vi "Init Range Single.vi"(8 "error in (no error)":errorcluster, 11 "Grove Ranging Sensor VL53L0X in":refnum<class "Grove Range Sensor VL53L0X .lvclass">) -> (0 "error out":errorcluster, 3 "Grove Ranging Sensor VL53L0X out":refnum<class "Grove Range Sensor VL53L0X .lvclass">)   [LabVIEW 2020, in "CTI-Peripheral.lvlib" / "Grove Range Sensor VL53L0X .lvclass"]
uses:
  Grove Range Sensor VL53L0X .lvclass
  Range Mode.ctl
  Sensor Command.ctl
  Registers.ctl
  Grove Range Sensor VL53L0X .lvclass/Grove Range Sensor VL53L0X .ctl
  CTI/I2C Connection/I2C Connection.lvclass/I2C Connection.ctl
  CTI/Session/I2C Write Data.vi
  CTI/Session/I2C Read Data.vi
  CTI/I2C Connection/I2C Connection.lvclass
panel:
  out "Init Data":string
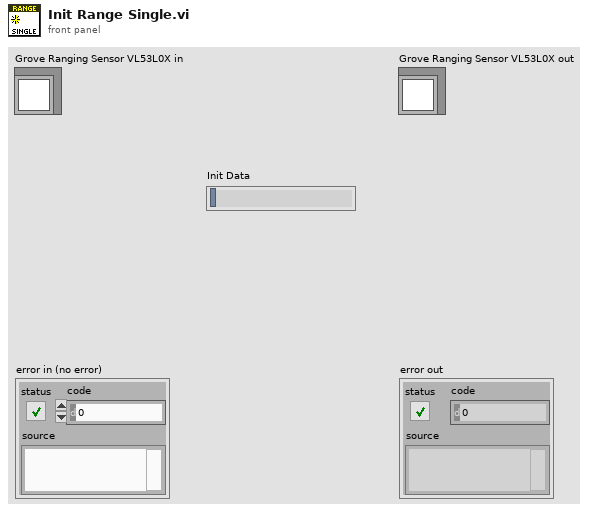
[diagram p1: front panel]
types:
  T1 = typedef "CTI-Peripheral.lvlib/Grove Range Sensor VL53L0X .lvclass/Sensor Command.ctl" = cluster{"Registers":T2, "Data":u8[], "ReadBack Len":u8}
  T2 = typedef "CTI-Peripheral.lvlib/Grove Range Sensor VL53L0X .lvclass/Registers.ctl" = u16
  T3 = typedef "CTI-Peripheral.lvlib/Grove Range Sensor VL53L0X .lvclass/Range Mode.ctl" = enum16{"No Mode - Error", "Single", "Continuous", "High Speed", "High Accuracy", "Long Distance"}
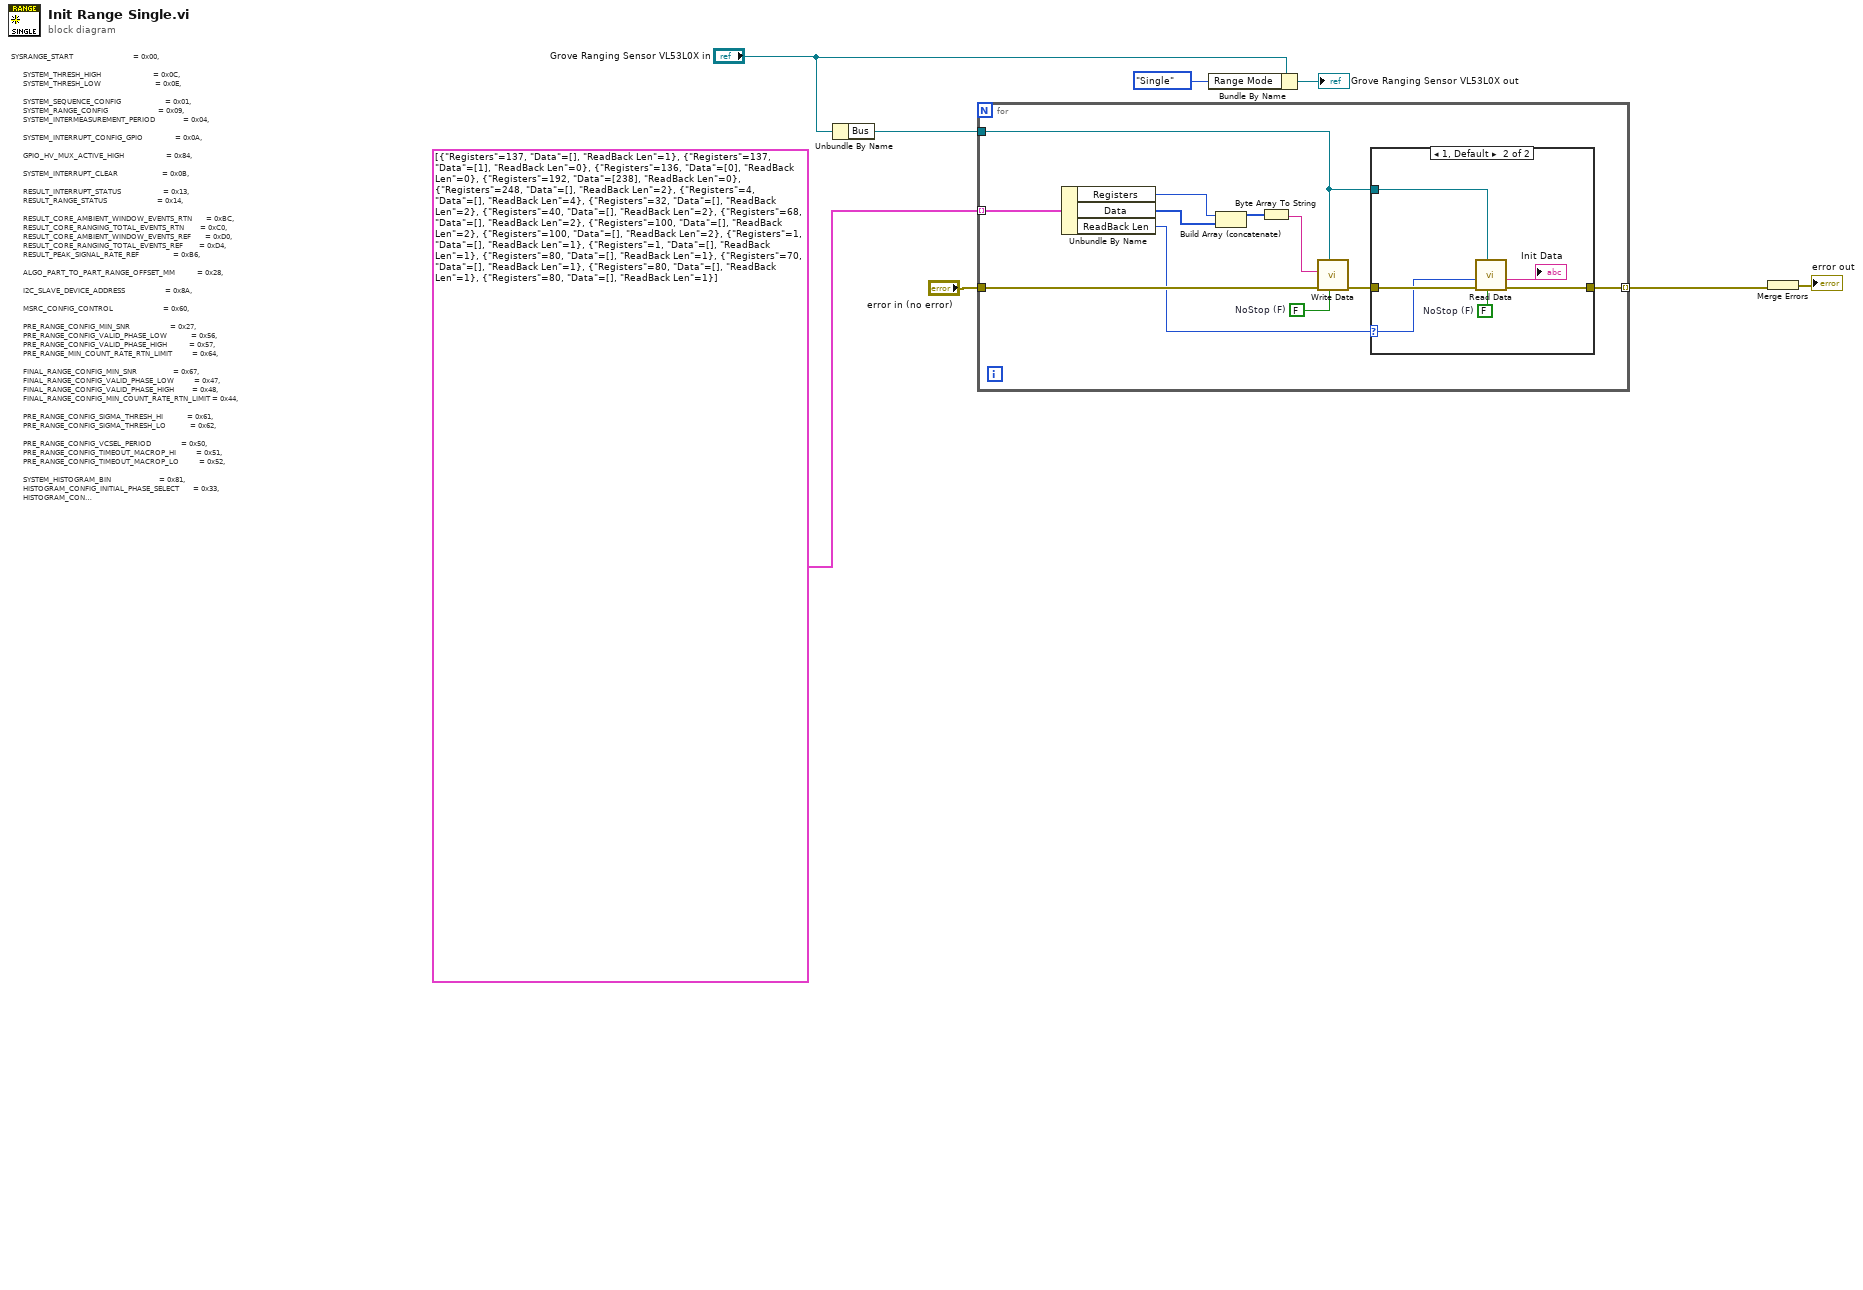
[diagram p0: block diagram]
diagram:
  # "SYSRANGE_START                              = 0x00,\n\n      SYSTEM_THRESH_HIGH                          = 0x0C,\n      SYSTEM_THRESH_LOW                           = 0x0E,\n\n      SYSTEM_SEQUENCE_CONFIG                      = 0x01,\n      SYSTEM_RANGE_CONFIG                         = 0x09,\n      SYSTEM_INTERMEASUREMENT_PERIOD              = 0x04,\n\n      SYSTEM_INTERRUPT_CONFIG_GPIO                = 0x0A,\n\n      GPIO_HV_MUX_ACTIVE_HIGH                     = 0x84,\n\n      SYSTEM_INTERRUPT_CLEAR                      = 0x0B,\n\n      RESULT_INTERRUPT_STATUS                     = 0x13,\n      RESULT_RANGE_STATUS                         = 0x14,\n\n      RESULT_CORE_AMBIENT_WINDOW_EVENTS_RTN       = 0xBC,\n      RESULT_CORE_RANGING_TOTAL_EVENTS_RTN        = 0xC0,\n      RESULT_CORE_AMBIENT_WINDOW_EVENTS_REF       = 0xD0,\n      RESULT_CORE_RANGING_TOTAL_EVENTS_REF        = 0xD4,\n      RESULT_PEAK_SIGNAL_RATE_REF                 = 0xB6,\n\n      ALGO_PART_TO_PART_RANGE_OFFSET_MM           = 0x28,\n\n      I2C_SLAVE_DEVICE_ADDRESS                    = 0x8A,\n\n      MSRC_CONFIG_CONTROL                         = 0x60,\n\n      PRE_RANGE_CONFIG_MIN_SNR                    = 0x27,\n      PRE_RANGE_CONFIG_VALID_PHASE_LOW            = 0x56,\n      PRE_RANGE_CONFIG_VALID_PHASE_HIGH           = 0x57,\n      PRE_RANGE_MIN_COUNT_RATE_RTN_LIMIT          = 0x64,\n\n      FINAL_RANGE_CONFIG_MIN_SNR                  = 0x67,\n      FINAL_RANGE_CONFIG_VALID_PHASE_LOW          = 0x47,\n      FINAL_RANGE_CONFIG_VALID_PHASE_HIGH         = 0x48,\n      FINAL_RANGE_CONFIG_MIN_COUNT_RATE_RTN_LIMIT = 0x44,\n\n      PRE_RANGE_CONFIG_SIGMA_THRESH_HI            = 0x61,\n      PRE_RANGE_CONFIG_SIGMA_THRESH_LO            = 0x62,\n\n      PRE_RANGE_CONFIG_VCSEL_PERIOD               = 0x50,\n      PRE_RANGE_CONFIG_TIMEOUT_MACROP_HI          = 0x51,\n      PRE_RANGE_CONFIG_TIMEOUT_MACROP_LO          = 0x52,\n\n      SYSTEM_HISTOGRAM_BIN                        = 0x81,\n      HISTOGRAM_CONFIG_INITIAL_PHASE_SELECT       = 0x33,\n      HISTOGRAM_CONFIG_READOUT_CTRL               = 0x55,\n\n      FINAL_RANGE_CONFIG_VCSEL_PERIOD             = 0x70,\n      FINAL_RANGE_CONFIG_TIMEOUT_MACROP_HI        = 0x71,\n      FINAL_RANGE_CONFIG_TIMEOUT_MACROP_LO        = 0x72,\n      CROSSTALK_COMPENSATION_PEAK_RATE_MCPS       = 0x20,\n\n      MSRC_CONFIG_TIMEOUT_MACROP                  = 0x46,\n\n      SOFT_RESET_GO2_SOFT_RESET_N                 = 0xBF,\n      IDENTIFICATION_MODEL_ID                     = 0xC0,\n      IDENTIFICATION_REVISION_ID                  = 0xC2,\n\n      OSC_CALIBRATE_VAL                           = 0xF8,\n\n      GLOBAL_CONFIG_VCSEL_WIDTH                   = 0x32,\n      GLOBAL_CONFIG_SPAD_ENABLES_REF_0            = 0xB0,\n      GLOBAL_CONFIG_SPAD_ENABLES_REF_1            = 0xB1,\n      GLOBAL_CONFIG_SPAD_ENABLES_REF_2            = 0xB2,\n      GLOBAL_CONFIG_SPAD_ENABLES_REF_3            = 0xB3,\n      GLOBAL_CONFIG_SPAD_ENABLES_REF_4            = 0xB4,\n      GLOBAL_CONFIG_SPAD_ENABLES_REF_5            = 0xB5,\n\n      GLOBAL_CONFIG_REF_EN_START_SELECT           = 0xB6,\n      DYNAMIC_SPAD_NUM_REQUESTED_REF_SPAD         = 0x4E,\n      DYNAMIC_SPAD_REF_EN_START_OFFSET            = 0x4F,\n      POWER_MANAGEMENT_GO1_POWER_FORCE            = 0x80,\n\n      VHV_CONFIG_PAD_SCL_SDA__EXTSUP_HV           = 0x89,\n\n      ALGO_PHASECAL_LIM                           = 0x30,\n      ALGO_PHASECAL_CONFIG_TIMEOUT                = 0x30,\n    };"
  n1 = Unbundle By Name("Grove Ranging Sensor VL53L0X in") -> ("Bus"=w8:refnum<class "I2C Connection.lvclass">)
  n2 = for {
    tunnel: w8 -> [w19]
    tunnel: "error in (no error)" -> [w15]
    tunnel: [w13] -> w2 mode=indexing
    tunnel: T1[] [{"Registers"=137, "Data"=[], "ReadBack Len"=1}, {"Registers"=137, "Data"=[1], "ReadBack Len"=0}, {"Registers"=136, "Data"=[0], "ReadBack Len"=0}, {"Registers"=192, "Data"=[238], "ReadBack Len"=0}, {"Registers"=248, "Data"=[], "ReadBack Len"=2}, {"Registers"=4, "Data"=[], "ReadBack Len"=4}, {"Registers"=32, "Data"=[], "ReadBack Len"=2}, {"Registers"=40, "Data"=[], "ReadBack Len"=2}, {"Registers"=68, "Data"=[], "ReadBack Len"=2}, {"Registers"=100, "Data"=[], "ReadBack Len"=2}, {"Registers"=100, "Data"=[], "ReadBack Len"=2}, {"Registers"=1, "Data"=[], "ReadBack Len"=1}, {"Registers"=1, "Data"=[], "ReadBack Len"=1}, {"Registers"=80, "Data"=[], "ReadBack Len"=1}, {"Registers"=70, "Data"=[], "ReadBack Len"=1}, {"Registers"=80, "Data"=[], "ReadBack Len"=1}, {"Registers"=80, "Data"=[], "ReadBack Len"=1}] -> [w12] mode=indexing
    w18 = FALSE  # NoStop (F)
    n3 = Unbundle By Name(w12) -> ("Registers"=w11:T2, "Data"=w10:u8[], "ReadBack Len"=w9:u8)
    n4 = Build Array (concatenate)(w11, w10) -> (w16:T2[])
    n5 = Byte Array To String(unsigned byte array=w16) -> (string=w17:string)
    n6 = call "Write Data.vi"("NoStop (F)"=w18, "I2C Connection"=w19, "error in (no error)"=w15, "Data"=w17) -> ("error out"=w14:errorcluster)  [unwired: 7 in]
    n7 = case shown="1, Default" w9 {
      selector: w9 -> [_ w21]
      tunnel: w19 -> [_ w26]
      tunnel: w14 -> [w20 w23]
      tunnel: [w20 w22] -> w13
      frame 0 {
      }
      frame 1, Default {
        w25 = FALSE  # NoStop (F)
        n8 = call "Read Data.vi"("NoStop (F)"=w25, "I2C Connection"=w26, "error in (no error)"=w23, "Len"=w21) -> ("error out"=w22:errorcluster, "Data"=→"Init Data":string)  [unwired: 6 in]
      }
    }
  }
  n9 = Bundle By Name(cluster="Grove Ranging Sensor VL53L0X in", "Range Mode"=Range_Mode."Single") -> (→"Grove Ranging Sensor VL53L0X out":refnum<class "Grove Range Sensor VL53L0X .lvclass">)
  n10 = Merge Errors(w2) -> (→"error out":errorcluster)
